vi "Get Datalogger.vi"(8 "error in (no error)":errorcluster, 11 "Sequencer in":refnum<class "Sequencer.lvclass">) -> (0 "error out":errorcluster, 3 "Datalogger":refnum<class "Datalogger.lvclass">)   [LabVIEW 2020]
uses:
  edb1111e-0500-4cb0-8859-1b29db90b009.vi
  Classes/Datalogger/Datalogger.lvclass
  Sequencer.lvclass
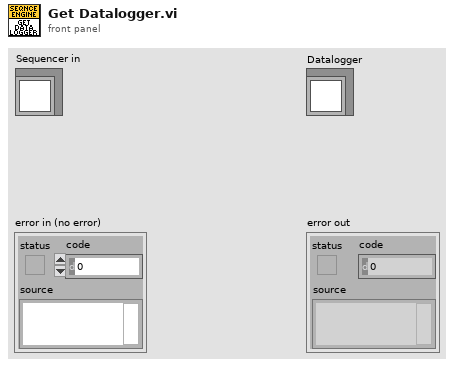
[diagram p1: front panel]
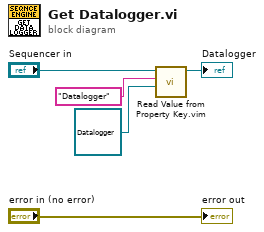
[diagram p0: block diagram]
diagram:
  n1 = call "Read Value from Property Key.vim"("Type"=refnum<class "Datalogger.lvclass"> refnum ("Datalogger"), "Key"="Datalogger", "Service in"="Sequencer in") -> ("Value"=→"Datalogger":refnum<class "Datalogger.lvclass">)  [unwired: 7 in, 1 out]
  "error out" <- "error in (no error)"
